vi "Player Info.vi"(11 "Atomic in":refnum<class "Atomic.lvclass">) -> (0 "Defeat Speech":string, 1 "Victory Speech":string, 2 "Name":string, 3 "Atomic out":refnum<class "Atomic.lvclass">)   [LabVIEW 2017, in "Atomic.lvclass"]
uses:
  Atomic.lvclass
  Square/Square.lvclass
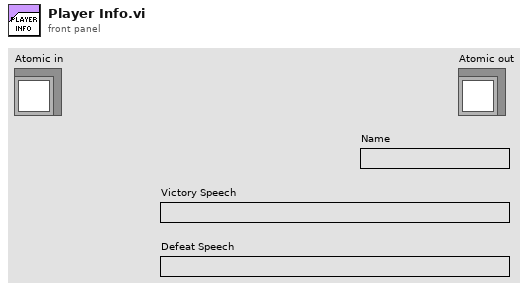
[diagram p1: front panel]
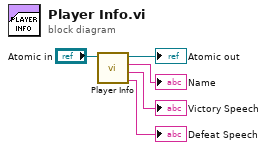
[diagram p0: block diagram]
diagram:
  n1 = call-parent "Player Info.vi"("Square in"="Atomic in") -> ("Defeat Speech"=→"Defeat Speech":string, "Victory Speech"=→"Victory Speech":string, "Name"=→"Name":string, "Square out"=→"Atomic out":refnum<class "Atomic.lvclass">)  [unwired: 7 in]
